vi "init_param_generator.vi"(1 "Limit":i16[](array[numeric]), 2 "Servo":i16[](array[numeric]), 3 "mag offset 2":i16, 4 "mag offset 1":i16, 6 "mode":enum16{"Manual", "Quad", "Vertical", "Half"}(ring)) -> (0 "init param":string)   [LabVIEW 2013]
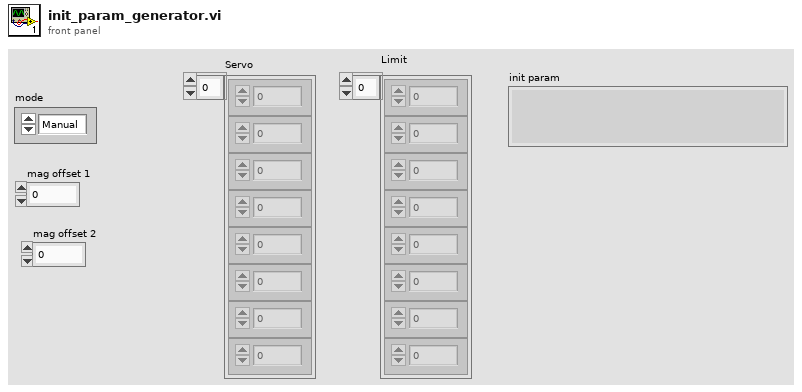
[diagram p1: front panel]
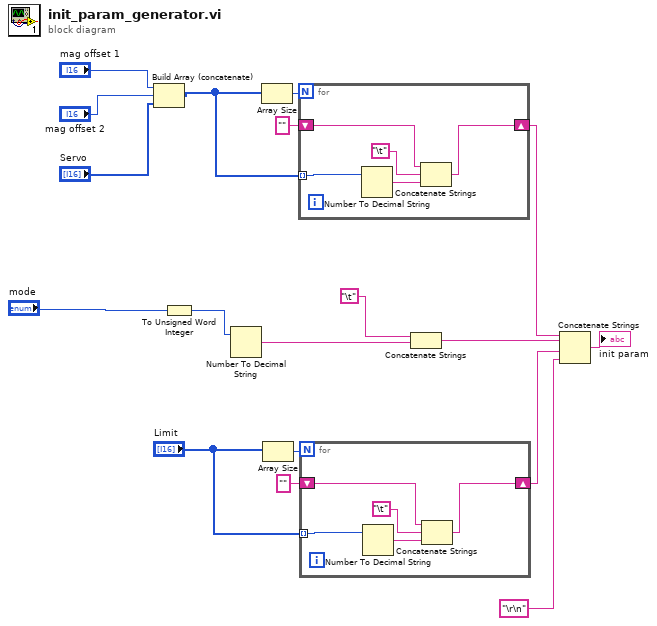
[diagram p0: block diagram]
diagram:
  n1 = Build Array (concatenate)("mag offset 1", "mag offset 2", "Servo") -> (w7:i16[])
  n2 = To Unsigned Word Integer(number="mode") -> (unsigned 16bit integer=w12:u16)
  n3 = Number To Decimal String(number=w12) -> (decimal integer string=w14:string)  [unwired: 1 in]
  n4 = Array Size(array=w7) -> (size(s)=w17:i32)
  n5 = Array Size(array="Limit") -> (size(s)=w6:i32)
  n6 = for {
    N: w17 -> [_]
    tunnel: w7 -> [w23] mode=indexing
    shift-right: [w20] -> w15
    shift-left: "" -> [w19]
    n7 = Number To Decimal String(number=w23) -> (decimal integer string=w21:string)  [unwired: 1 in]
    n8 = Concatenate Strings(w19, "\t", w21) -> (w20:string)
  }
  n9 = for {
    N: w6 -> [_]
    tunnel: "Limit" -> [w28] mode=indexing
    shift-right: [w25] -> w3
    shift-left: "" -> [w24]
    n10 = Number To Decimal String(number=w28) -> (decimal integer string=w26:string)  [unwired: 1 in]
    n11 = Concatenate Strings(w24, "\t", w26) -> (w25:string)
  }
  n12 = Concatenate Strings("\t", w14) -> (w16:string)
  n13 = Concatenate Strings(w15, w16, w3, "\r\n" ("ctr_buffer")) -> (→"init param":string)
